vi "3-lorentzian-heat-response -- analytic derivatives -- grad and curvature -- V4.vi"(6 "parameters map  IN":map{T1, dbl}(c390), 7 "action":T2=enum."d-all", 10 "ω (rad/sec)":dbl=0.1 format="%#_10f") -> (0 "second derivatives map out":map{i32[], cdb}(c390), 1 "grad map  out":map{i32, cdb}(c390), 2 "ω out (rad/sec)":dbl=0.1 format="%#_10f", 3 "R(ω)":cdb=0.1+0.0i format="%#_10f")   [LabVIEW 2020]
uses:
  3-lorentzian-heat-response action.ctl
  3-lorentzian-parameters.ctl
panel:
  in  "κ0":dbl(slide)=6.091279771876994e-09 min=0.0 max=0.3 step=1e-12 scale=1e-10..1e-06 scale format="%#_3p"
  in  "ζ":dbl(slide)=0.016395386176563286 min=0.0 max=0.3 step=1e-06 scale=1e-05..1000.0 scale format="%#_3p"
  in  "τN":dbl(slide)=0.0007964886373917906 min=0.0 max=0.3 step=1e-06 scale=1e-06..10.0 scale format="%#_3p"
  in  "T1":dbl(slide)=0.017784241145719432 min=0.0 max=0.3 step=1e-06 scale=0.0001..10.0 scale format="%#_3p"
  in  "τC":dbl(slide)=0.0055481925503790405 min=0.0 max=0.3 step=1e-06 scale=0.0001..10.0 scale format="%#_3p"
  in  "τS":dbl(slide)=0.01833817297436167 min=0.0 max=0.3 step=1e-06 scale=0.0001..10.0 scale format="%#_3p"
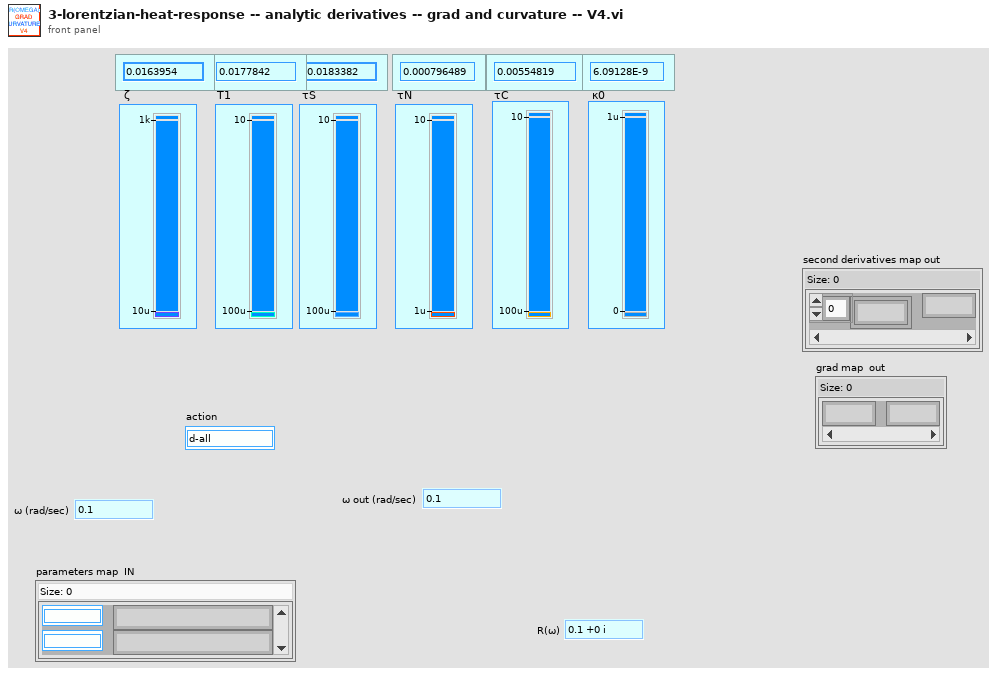
[diagram p1: front panel]
types:
  T1 = typedef "3-lorentzian-parameters.ctl" = enum16{"ζ", "τ1", "τS", "τN", "τC", "κ0", "m1", "m2", "m3", "T (K)", "B (T)", "θ (deg)", "side (S|R)", "set of (B|T)"}
  T2 = typedef "3-lorentzian-heat-response action.ctl" = enum16{"calc R", "create string", "calc m1m2m3", "dζ", "dT1", "dτS", "dτN", "dτC", "d-all", "dκ0", "T(K)", "m1", "m2", "m3", "parse string", "θ (deg)", "B (T)", "onlygrads", "newton", "create emty string"}
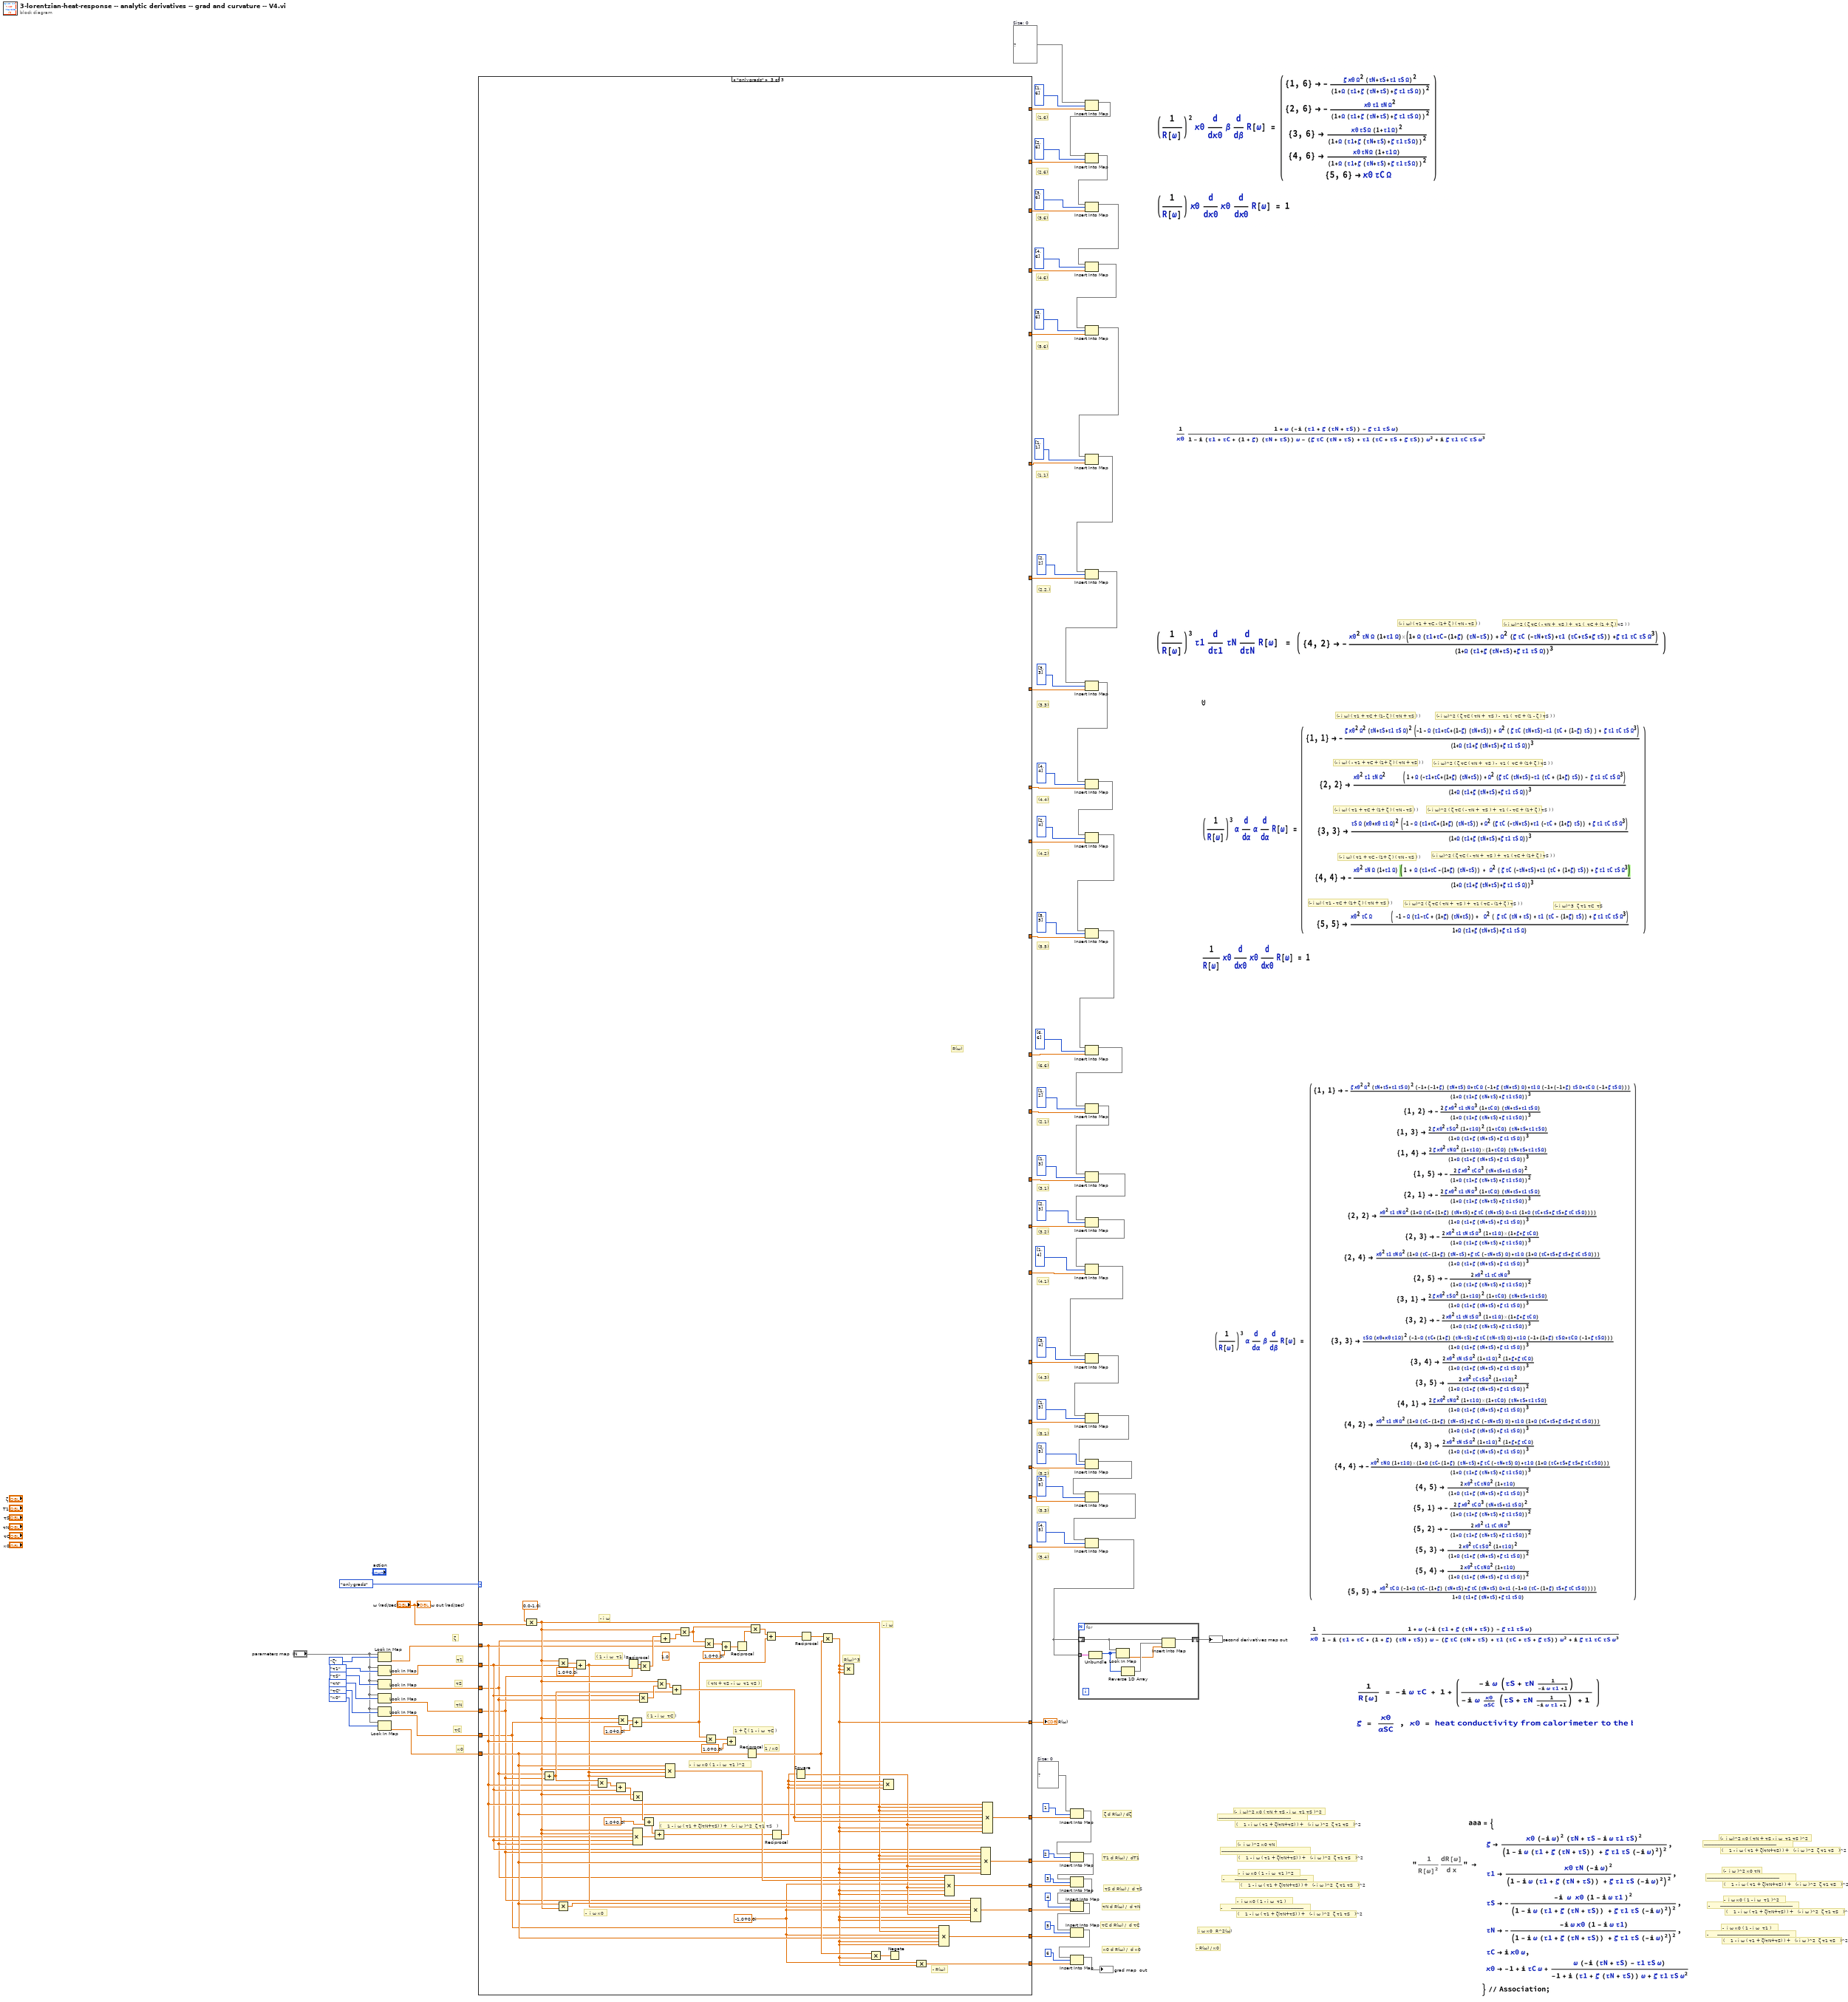
[diagram p0: block diagram]
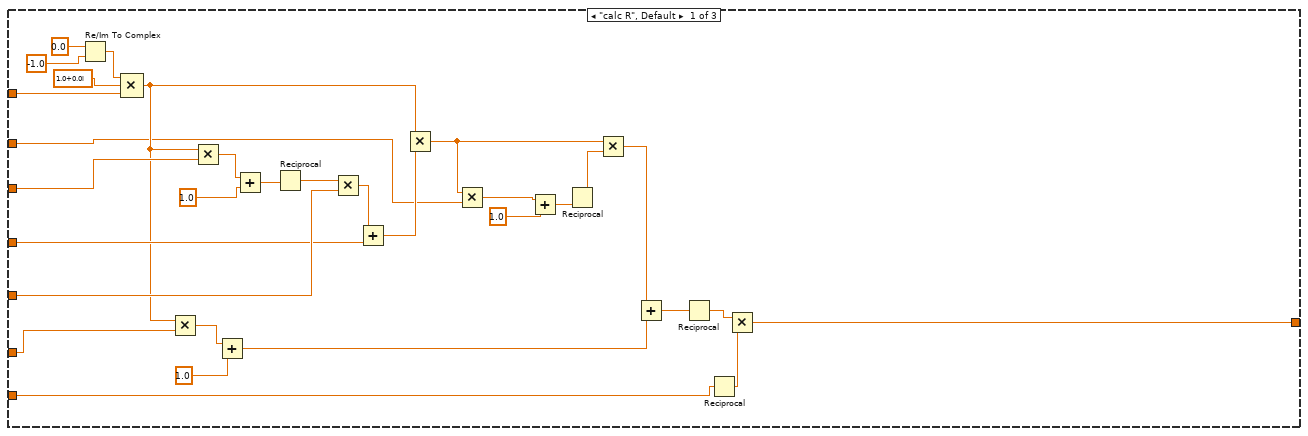
[diagram p2: hidden frame]
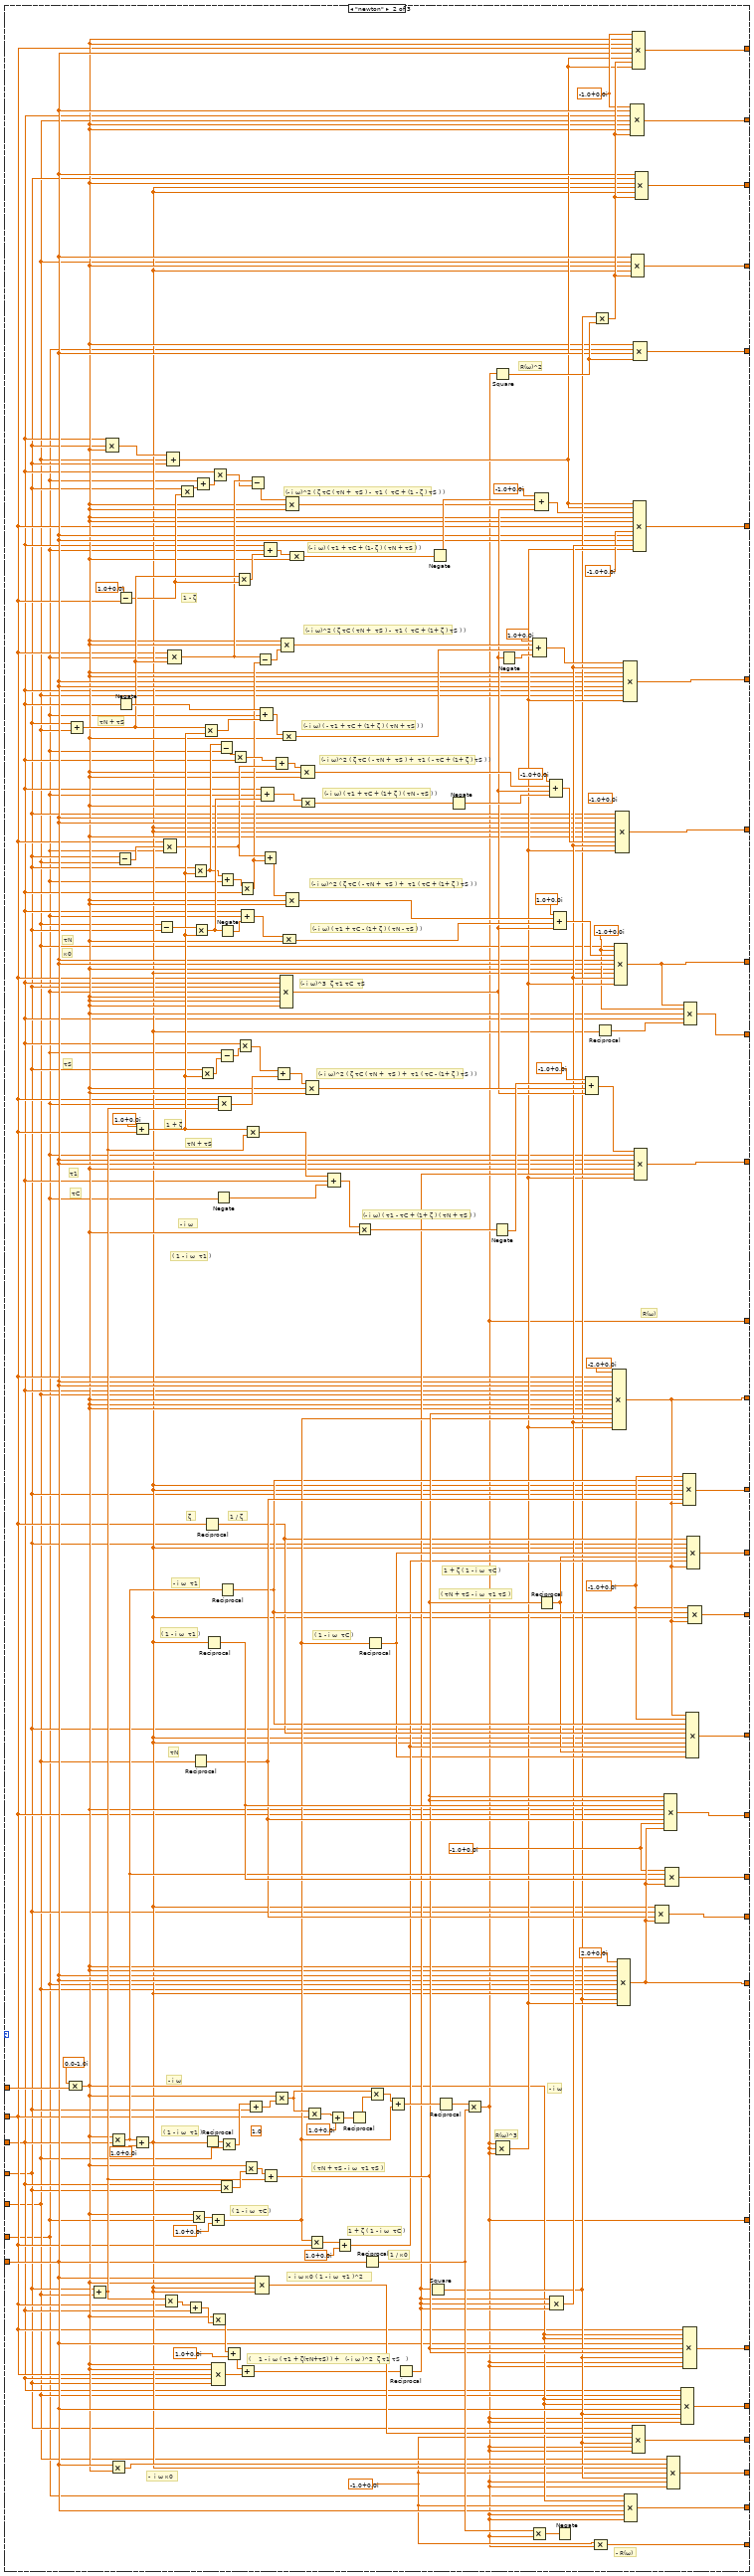
[diagram p3: hidden frame]
diagram:
  w27 = map{i32, cdb} {}  # Size: 0
  w85 = map{i32[], cdb} {}  # Size: 0
  # "κ0 d R(ω) /  d κ0"
  # "τC d R(ω) /  d τC"
  # "τN d R(ω) /  d τN"
  # "τS d R(ω) /  d τS"
  # "T1 d R(ω) /  dT1"
  # "ζ d R(ω) / dζ"
  # "(4,2)"
  # "(- i ω)^2 ( ζ τC ( - τN +  τS ) +  τ1 (  τC + (1 + ζ ) τS ) )"
  # "(- i ω) ( τ1 + τC - (1+ ζ ) ( τN - τS ) )"
  # "(1,6)"
  # "(2,6)"
  # "(3,6)"
  # "(4,6)"
  # "(5,6)"
  # "(1,1)"
  # "(- i ω)^2 ( ζ τC ( τN +  τS ) -  τ1 (  τC + (1 - ζ ) τS ) )"
  # "(- i ω) ( τ1 + τC + (1- ζ ) ( τN + τS ) )"
  # "(2,2,)"
  # "(- i ω)^2 ( ζ τC ( τN +  τS ) -  τ1 (  τC + (1+ ζ ) τS ) )"
  # "(- i ω) ( - τ1 + τC + (1+ ζ ) ( τN + τS ) )"
  # "(3,3)"
  # "(- i ω)^2 ( ζ τC ( - τN +  τS ) +  τ1 ( - τC + (1+ ζ ) τS ) )"
  # "(- i ω) ( τ1 + τC + (1+ ζ ) ( τN - τS ) )"
  # "(4,4)"
  # "(- i ω)^2 ( ζ τC ( - τN +  τS ) +  τ1 ( τC + (1+ ζ ) τS ) )"
  # "(- i ω) ( τ1 + τC - (1+ ζ ) ( τN - τS ) )"
  # "(- i ω)^3  ζ τ1 τC  τS"
  # "(- i ω) ( τ1 - τC + (1+ ζ ) ( τN + τS ) )"
  # "(- i ω)^2 ( ζ τC ( τN +  τS ) +  τ1 ( τC - (1+ ζ ) τS ) )"
  # "(5,5)"
  # "(6,6)"
  # "(4,3)"
  # "(4,1)"
  # "(3,2)"
  # "(3,1)"
  # "(2,1)"
  # "(5,1)"
  # "(5,2)"
  # "(5,3)"
  # "κ0"
  # "τC"
  # "τN"
  # "τS"
  # "τ1"
  # "ζ"
  # "(5,4)"
  # "-------------------------------------------------"
  # "(-  i ω)^2 κ0 ( τN + τS - i ω  τ1 τS )^2"
  # "(    1 - i ω ( τ1 + ζ(τN+τS) ) +   (- i ω )^2  ζ τ1 τS   )^2"
  # "-------------------------------------------------"
  # "(-  i ω )^2 κ0 τN"
  # "(    1 - i ω ( τ1 + ζ(τN+τS) ) +   (- i ω )^2  ζ τ1 τS   )^2"
  # "-      -------------------------------------------------"
  # "-  i ω κ0 ( 1 - i ω  τ1 )"
  # "(    1 - i ω ( τ1 + ζ(τN+τS) ) +   (- i ω )^2  ζ τ1 τS   )^2"
  # "-       -------------------------------------------------"
  # "-  i ω κ0 ( 1 - i ω  τ1 )^2"
  # "(    1 - i ω ( τ1 + ζ(τN+τS) ) +   (- i ω )^2  ζ τ1 τS   )^2"
  # "-------------------------------------------------"
  # "(-  i ω)^2 κ0 ( τN + τS - i ω  τ1 τS )^2"
  # "(    1 - i ω ( τ1 + ζ(τN+τS) ) +   (- i ω )^2  ζ τ1 τS   )^2"
  # "-------------------------------------------------"
  # "(-  i ω )^2 κ0 τN"
  # "(    1 - i ω ( τ1 + ζ(τN+τS) ) +   (- i ω )^2  ζ τ1 τS   )^2"
  # "-      -------------------------------------------------"
  # "-  i ω κ0 ( 1 - i ω  τ1 )"
  # "(    1 - i ω ( τ1 + ζ(τN+τS) ) +   (- i ω )^2  ζ τ1 τS   )^2"
  # "-       -------------------------------------------------"
  # "-  i ω κ0 ( 1 - i ω  τ1 )^2"
  # "(    1 - i ω ( τ1 + ζ(τN+τS) ) +   (- i ω )^2  ζ τ1 τS   )^2"
  # "i ω κ0  R^2(ω)"
  # "- R(ω) / κ0"
  n1 = Look In Map(map="parameters map  IN", key=3-lorentzian-parameters."ζ" ("Plost: sweep window")) -> (value=w91:dbl)  [unwired: 1 in, 1 out]
  n2 = Look In Map(map="parameters map  IN", key=3-lorentzian-parameters."τ1" ("Plost: sweep window")) -> (value=w90:dbl)  [unwired: 1 in, 1 out]
  n3 = Look In Map(map="parameters map  IN", key=3-lorentzian-parameters."τS" ("Plost: sweep window")) -> (value=w89:dbl)  [unwired: 1 in, 1 out]
  n4 = Look In Map(map="parameters map  IN", key=3-lorentzian-parameters."τN" ("Plost: sweep window")) -> (value=w88:dbl)  [unwired: 1 in, 1 out]
  n5 = Look In Map(map="parameters map  IN", key=3-lorentzian-parameters."τC" ("Plost: sweep window")) -> (value=w87:dbl)  [unwired: 1 in, 1 out]
  n6 = Look In Map(map="parameters map  IN", key=3-lorentzian-parameters."κ0" ("Plost: sweep window")) -> (value=w86:dbl)  [unwired: 1 in, 1 out]
  n7 = case shown="\"onlygrads\"" 3-lorentzian-heat-response_action."onlygrads" ("action") {
    tunnel: w87 -> [w117 w132 w289]
    tunnel: "ω (rad/sec)" -> [w120 w286 w339]
    tunnel: w90 -> [w119 w138 w295]
    tunnel: w88 -> [w125 w136 w293]
    tunnel: w89 -> [w123 w137 w294]
    tunnel: w91 -> [w113 w139 w296]
    tunnel: [w101 w134 w291] -> w100
    tunnel: w86 -> [w104 w148 w299]
    tunnel: [_ w133 w290] -> w10
    tunnel: [_ w274 w327] -> w14
    tunnel: [_ w263 w316] -> w20
    tunnel: [_ w261 w314] -> w16
    tunnel: [_ w260 w313] -> w23
    tunnel: [_ w257 w310] -> w25
    tunnel: [_ w251 _] -> w29
    tunnel: [_ w254 _] -> w31
    tunnel: [_ w253 _] -> w34
    tunnel: [_ w252 _] -> w37
    tunnel: [_ w237 _] -> w52
    tunnel: [_ w244 _] -> w49
    tunnel: [_ w239 _] -> w46
    tunnel: [_ w238 _] -> w43
    tunnel: [_ w236 _] -> w40
    tunnel: [_ w134 _] -> w56
    tunnel: [_ w214 _] -> w58
    tunnel: [_ w145 _] -> w60
    tunnel: [_ w194 _] -> w63
    tunnel: [_ w184 _] -> w66
    tunnel: [_ w160 _] -> w69
    tunnel: [_ w156 _] -> w71
    tunnel: [_ w153 _] -> w74
    tunnel: [_ w152 _] -> w78
    tunnel: [_ w151 _] -> w80
    tunnel: [_ w147 _] -> w83
    tunnel: [_ w140 _] -> w3
    frame "calc R", Default {
      n8 = Re/Im To Complex(1:-1.0 ("y"), 2:0.0 ("x")) -> (0:w121:cdb)
      n9 = Compound Arithmetic op=MULTIPLY(w121, cdb 1.0+0.0i ("value"), w120) -> (w115:cdb)
      n10 = Multiply(x=w115, y=w117) -> (x*y=w116:cdb)
      n11 = Multiply(x=w115, y=w119) -> (x*y=w118:cdb)
      n12 = Add(x=w116, y=1.0) -> (x+y=w107:cdb)
      n13 = Add(x=w118, y=1.0) -> (x+y=w127:cdb)
      n14 = Reciprocal(x=w127) -> (1/x=w126:cdb)
      n15 = Multiply(x=w126, y=w125) -> (x*y=w124:cdb)
      n16 = Add(x=w124, y=w123) -> (x+y=w114:cdb)
      n17 = Multiply(x=w115, y=w114) -> (x*y=w109:cdb)
      n18 = Multiply(x=w109, y=w113) -> (x*y=w111:cdb)
      n19 = Add(x=w111, y=1.0) -> (x+y=w110:cdb)
      n20 = Reciprocal(x=w110) -> (1/x=w108:cdb)
      n21 = Multiply(x=w109, y=w108) -> (x*y=w106:cdb)
      n22 = Add(x=w106, y=w107) -> (x+y=w105:cdb)
      n23 = Reciprocal(x=w105) -> (1/x=w103:cdb)
      n24 = Reciprocal(x=w104) -> (1/x=w102:dbl)
      n25 = Multiply(x=w103, y=w102) -> (x*y=w101:cdb)
    }
    frame "newton" {
      w149 = cdb -1.0+0.0i ("value")
      (unwired) cdb -1.0+0.0i ("value")
      w144 = cdb -1.0+0.0i ("value")
      w235 = cdb -1.0+0.0i ("value")
      w250 = cdb -1.0+0.0i ("value")
      w135 = cdb -1.0+0.0i ("value")
      (unwired) 1.0
      # "(- i ω)^2 ( ζ τC ( τN +  τS ) -  τ1 (  τC + (1 - ζ ) τS ) )"
      # "(- i ω) ( τ1 + τC + (1- ζ ) ( τN + τS ) )"
      # "τN + τS"
      # "(- i ω)^2 ( ζ τC ( τN +  τS ) -  τ1 (  τC + (1+ ζ ) τS ) )"
      # "(- i ω) ( - τ1 + τC + (1+ ζ ) ( τN + τS ) )"
      # "(- i ω)^2 ( ζ τC ( - τN +  τS ) +  τ1 ( - τC + (1+ ζ ) τS ) )"
      # "(- i ω) ( τ1 + τC + (1+ ζ ) ( τN - τS ) )"
      # "κ0"
      # "τN"
      # "( 1 - i ω  τ1 )"
      # "(- i ω)^2 ( ζ τC ( - τN +  τS ) +  τ1 ( τC + (1+ ζ ) τS ) )"
      # "(- i ω) ( τ1 + τC - (1+ ζ ) ( τN - τS ) )"
      # "τS"
      # "τ1"
      # "(- i ω)^3  ζ τ1 τC  τS"
      # "(- i ω)^2 ( ζ τC ( τN +  τS ) +  τ1 ( τC - (1+ ζ ) τS ) )"
      # "1 - ζ"
      # "(- i ω) ( τ1 - τC + (1+ ζ ) ( τN + τS ) )"
      # "- i ω"
      # "τC"
      # "τN + τS"
      # "1 + ζ"
      # "R(ω)"
      # "τN"
      # "1 / ζ"
      # "ζ"
      # "- i ω  τ1"
      # "( 1 - i ω  τ1 )"
      # "( τN + τS - i ω  τ1 τS )"
      # "1 + ζ ( 1 - i ω  τC )"
      # "( 1 - i ω  τC )"
      # "1 + ζ ( 1 - i ω  τC )"
      # "( 1 - i ω  τC )"
      # "R(ω)^3"
      # "( τN + τS - i ω  τ1 τS )"
      # "-  i ω κ0"
      # "( 1 - i ω  τ1 )"
      # "(    1 - i ω ( τ1 + ζ(τN+τS) ) +   (- i ω )^2  ζ τ1 τS   )"
      # "-  i ω κ0 ( 1 - i ω  τ1 )^2"
      # "- i ω"
      # "1 / κ0"
      # "- R(ω)"
      # "- i ω"
      # "R(ω)^2"
      n26 = Add(x=w137, y=w136) -> (x+y=w182:dbl)
      n27 = Compound Arithmetic op=MULTIPLY(cdb 0.0-1.0i ("value"), w286) -> (w143:cdb)
      n28 = Add(x=w137, y=w136) -> (x+y=w225:dbl)
      n29 = Compound Arithmetic op=MULTIPLY(w138, w137, w143) -> (w159:cdb)
      n30 = Multiply(x=w143, y=w138) -> (x*y=w246:cdb)
      n31 = Multiply(x=w148, y=w143) -> (x*y=w262:cdb)
      n32 = Subtract(x=w137, y=w136) -> (x-y=w209:dbl)
      n33 = Subtract(x=cdb 1.0+0.0i ("value"), y=w139) -> (x-y=w173:cdb)
      n34 = Negate(x=w138) -> (-x=w192:dbl)
      n35 = Add(x=cdb 1.0+0.0i ("value"), y=w139) -> (x+y=w193:cdb)
      n36 = Add(x=w246, y=cdb 1.0+0.0i ("value")) -> (x+y=w142:cdb)
      n37 = Subtract(x=w136, y=w137) -> (x-y=w212:dbl)
      n38 = Multiply(x=w225, y=w139) -> (x*y=w270:dbl)
      n39 = Compound Arithmetic op=MULTIPLY(w139, w209, w132) -> (w200:dbl)
      n40 = Compound Arithmetic op=ADD(w159, w136, w137) -> (w146:cdb)
      n41 = Compound Arithmetic op=MULTIPLY(w139, w132, w182) -> (w170:dbl)
      n42 = Multiply(x=w137, y=w173) -> (x*y=w172:cdb)
      n43 = Add(x=w270, y=w138) -> (x+y=w269:dbl)
      n44 = Multiply(x=w143, y=w132) -> (x*y=w285:cdb)
      n45 = Multiply(x=w137, y=w193) -> (x*y=w203:cdb)
      n46 = Reciprocal(x=w136) -> (1/x=w245:dbl)
      n47 = Multiply(x=w212, y=w193) -> (x*y=w204:cdb)
      n48 = Add(x=w132, y=w172) -> (x+y=w171:cdb)
      n49 = Multiply(x=w137, y=w193) -> (x*y=w224:cdb)
      n50 = Multiply(x=w182, y=w193) -> (x*y=w191:cdb)
      n51 = Reciprocal(x=w139) -> (1/x=w233:dbl)
      n52 = Reciprocal(x=w142) -> (1/x=w288:cdb)
      n53 = Reciprocal(x=w142) -> (1/x=w247:cdb)
      n54 = Add(x=w285, y=cdb 1.0+0.0i ("value")) -> (x+y=w242:cdb)
      n55 = Multiply(x=w143, y=w269) -> (x*y=w268:cdb)
      n56 = Multiply(x=w138, y=w171) -> (x*y=w169:cdb)
      n57 = Compound Arithmetic op=MULTIPLY(w143, w143, w139, w138, w137) -> (w265:cdb)
      n58 = Negate(x=w132) -> (-x=w228:dbl)
      n59 = Subtract(x=w203, y=w132) -> (x-y=w202:cdb)
      n60 = Multiply(x=w138, y=w137) -> (x*y=w259:dbl)
      n61 = Subtract(x=w132, y=w224) -> (x-y=w223:cdb)
      n62 = Compound Arithmetic op=MULTIPLY(w139, w132, w225) -> (w221:dbl)
      n63 = Add(x=w203, y=w132) -> (x+y=w210:cdb)
      n64 = Negate(x=w204) -> (-x=w211:cdb)
      n65 = Reciprocal(x=w246) -> (1/x=w234:cdb)
      n66 = Multiply(x=w288, y=w136) -> (x*y=w287:cdb)
      n67 = Add(x=w268, y=cdb 1.0+0.0i ("value")) -> (x+y=w266:cdb)
      n68 = Multiply(x=w202, y=w138) -> (x*y=w201:cdb)
      n69 = Multiply(x=w182, y=w173) -> (x*y=w181:cdb)
      n70 = Multiply(x=w138, y=w223) -> (x*y=w222:cdb)
      n71 = Multiply(x=w210, y=w138) -> (x*y=w189:cdb)
      n72 = Add(x=w266, y=w265) -> (x+y=w248:cdb)
      n73 = Compound Arithmetic op=ADD(w138, w132, w211) -> (w175:cdb)
      n74 = Multiply(x=w143, y=w259) -> (x*y=w258:cdb)
      n75 = Multiply(x=w193, y=w225) -> (x*y=w229:cdb)
      n76 = Add(x=w287, y=w137) -> (x+y=w284:cdb)
      n77 = Subtract(x=w170, y=w169) -> (x-y=w168:cdb)
      n78 = Compound Arithmetic op=MULTIPLY(w148, w143, w142, w142) -> (w264:cdb)
      n79 = Subtract(x=w170, y=w189) -> (x-y=w179:cdb)
      n80 = Compound Arithmetic op=ADD(w192, w132, w191) -> (w190:cdb)
      n81 = Compound Arithmetic op=ADD(w138, w132, w204) -> (w177:cdb)
      n82 = Add(x=w200, y=w189) -> (x+y=w208:cdb)
      n83 = Add(x=w258, y=w225) -> (x+y=w243:cdb)
      n84 = Compound Arithmetic op=ADD(w138, w132, w181) -> (w180:cdb)
      n85 = Add(x=w201, y=w200) -> (x+y=w199:cdb)
      n86 = Multiply(x=w143, y=w284) -> (x*y=w281:cdb)
      n87 = Add(x=w222, y=w221) -> (x+y=w220:cdb)
      n88 = Compound Arithmetic op=MULTIPLY(w139, w138, w137, w132, w143, w143, w143) -> (w163:cdb)
      n89 = Compound Arithmetic op=MULTIPLY(w143, w143, w179) -> (w178:cdb)
      n90 = Compound Arithmetic op=MULTIPLY(w190, w143) -> (w187:cdb)
      n91 = Compound Arithmetic op=MULTIPLY(w175, w143) -> (w174:cdb)
      n92 = Compound Arithmetic op=MULTIPLY(w168, w143, w143) -> (w164:cdb)
      n93 = Compound Arithmetic op=MULTIPLY(w208, w143, w143) -> (w206:cdb)
      n94 = Compound Arithmetic op=MULTIPLY(w180, w143) -> (w166:cdb)
      n95 = Compound Arithmetic op=MULTIPLY(w199, w143, w143) -> (w197:cdb)
      n96 = Compound Arithmetic op=MULTIPLY(w177, w143) -> (w176:cdb)
      n97 = Compound Arithmetic op=MULTIPLY(w220, w143, w143) -> (w216:cdb)
      n98 = Multiply(x=w281, y=w139) -> (x*y=w283:cdb)
      n99 = Multiply(x=w242, y=w139) -> (x*y=w241:cdb)
      n100 = Compound Arithmetic op=ADD(w229, w138, w228) -> (w227:cdb)
      n101 = Add(x=w283, y=cdb 1.0+0.0i ("value")) -> (x+y=w282:cdb)
      n102 = Add(x=w241, y=cdb 1.0+0.0i ("value")) -> (x+y=w232:cdb)
      n103 = Reciprocal(x=w282) -> (1/x=w280:cdb)
      n104 = Multiply(x=w227, y=w143) -> (x*y=w219:cdb)
      n105 = Reciprocal(x=w148) -> (1/x=w276:dbl)
      n106 = Reciprocal(x=w242) -> (1/x=w230:cdb)
      n107 = Multiply(x=w281, y=w280) -> (x*y=w279:cdb)
      n108 = Add(x=w279, y=w242) -> (x+y=w278:cdb)
      n109 = Reciprocal(x=w248) -> (1/x=w213:cdb)
      n110 = Square(x=w213) -> (x^2=w154:cdb)
      n111 = Negate(x=w166) -> (-x=w165:cdb)
      n112 = Reciprocal(x=w278) -> (1/x=w277:cdb)
      n113 = Negate(x=w176) -> (-x=w196:cdb)
      n114 = Multiply(x=w277, y=w276) -> (x*y=w134:cdb)
      n115 = Negate(x=w219) -> (-x=w217:cdb)
      n116 = Square(x=w134) -> (x^2=w155:cdb)
      n117 = Compound Arithmetic op=MULTIPLY(w134, w134, w134) -> (w157:cdb)
      n118 = Negate(x=w163) -> (-x=w186:cdb)
      n119 = Multiply(x=w276, y=w134) -> (x*y=w275:cdb)
      n120 = Compound Arithmetic op=ADD(cdb 1.0+0.0i ("value"), w178, w187, w186) -> (w185:cdb)
      n121 = Compound Arithmetic op=ADD(cdb -1.0+0.0i ("value"), w165, w164, w163) -> (w162:cdb)
      n122 = Reciprocal(x=w243) -> (1/x=w231:cdb)
      n123 = Compound Arithmetic op=ADD(cdb -1.0+0.0i ("value"), w197, w163, w196) -> (w195:cdb)
      n124 = Compound Arithmetic op=MULTIPLY(w213, w213, w213) -> (w161:cdb)
      n125 = Compound Arithmetic op=ADD(cdb 1.0+0.0i ("value"), w206, w174, w163) -> (w205:cdb)
      n126 = Negate(x=w275) -> ()  [unwired: 1 out]
      n127 = Compound Arithmetic op=ADD(cdb -1.0+0.0i ("value"), w217, w216, w163) -> (w215:cdb)
      n128 = Multiply(x=w154, y=w155) -> (x*y=w150:cdb)
      n129 = Compound Arithmetic op=MULTIPLY(w135, w134) -> (w133:cdb)
      n130 = Reciprocal(x=w142) -> (1/x=w141:cdb)
      n131 = Compound Arithmetic op=MULTIPLY(cdb -2.0+0.0i ("value"), w139, w148, w148, w138, w136, w143, w143, w143, w243, w242, w161, w157) -> (w237:cdb)
      n132 = Compound Arithmetic op=MULTIPLY(w136, w144, w205, w148, w148, w143, w142, w161, w157) -> (w145:cdb)
      n133 = Compound Arithmetic op=MULTIPLY(w137, w148, w148, w142, w142, w143, w195, w161, w157) -> (w194:cdb)
      n134 = Compound Arithmetic op=MULTIPLY(cdb 2.0+0.0i ("value"), w143, w143, w148, w148, w132, w136, w142, w154, w157) -> (w251:cdb)
      n135 = Compound Arithmetic op=MULTIPLY(w185, w161, w143, w143, w148, w148, w138, w136, w157) -> (w184:cdb)
      n136 = Compound Arithmetic op=MULTIPLY(w132, w143, w135, w148, w134, w134) -> (w274:cdb)
      n137 = Compound Arithmetic op=MULTIPLY(w149, w148, w138, w136, w143, w143, w150) -> (w151:cdb)
      n138 = Compound Arithmetic op=MULTIPLY(w148, w136, w143, w142, w150) -> (w153:cdb)
      n139 = Compound Arithmetic op=MULTIPLY(w149, w143, w143, w139, w148, w146, w150, w146) -> (w147:cdb)
      n140 = Compound Arithmetic op=MULTIPLY(w137, w264, w135, w154, w134, w134) -> (w263:cdb)
      n141 = Compound Arithmetic op=MULTIPLY(w146, w146, w162, w143, w143, w139, cdb -1.0+0.0i ("value"), w148, w148, w161, w157) -> (w160:cdb)
      n142 = Compound Arithmetic op=MULTIPLY(w143, w132, w148, w155) -> (w156:cdb)
      n143 = Compound Arithmetic op=MULTIPLY(w215, w132, w148, w148, w143, w213, w157) -> (w214:cdb)
      n144 = Compound Arithmetic op=MULTIPLY(w148, w137, w143, w142, w142, w150) -> (w152:cdb)
      n145 = Compound Arithmetic op=MULTIPLY(w142, w137, w245, w251) -> (w254:cdb)
      n146 = Compound Arithmetic op=MULTIPLY(w243, w243, w247, w143, w139, w245, w250, w251) -> (w252:cdb)
      n147 = Compound Arithmetic op=MULTIPLY(w250, w246, w247, w251) -> (w253:cdb)
      n148 = Compound Arithmetic op=MULTIPLY(w136, w262, w142, w135, w154, w134, w134) -> (w261:cdb)
      n149 = Compound Arithmetic op=MULTIPLY(w138, w136, w143, w143, w148, w154, w134, w134) -> (w260:cdb)
      n150 = Compound Arithmetic op=MULTIPLY(w235, w234, w142, w142, w137, w245, w237) -> (w244:cdb)
      n151 = Compound Arithmetic op=MULTIPLY(w139, w143, w143, w148, w243, w243, w154, w134, w134) -> (w257:cdb)
      n152 = Compound Arithmetic op=MULTIPLY(w145, w144, w143, w138, w141) -> (w140:cdb)
      n153 = Compound Arithmetic op=MULTIPLY(w237, w235, w234, w137, w233, w142, w142, w232, w231, w230) -> (w236:cdb)
      n154 = Compound Arithmetic op=MULTIPLY(w233, w137, w142, w230, w231, w232, w237) -> (w239:cdb)
      n155 = Compound Arithmetic op=MULTIPLY(w235, w234, w142, w237) -> (w238:cdb)
    }
    frame "onlygrads" {
      w292 = cdb -1.0+0.0i ("value")
      (unwired) 1.0
      # "R(ω)"
      # "1 + ζ ( 1 - i ω  τC )"
      # "( 1 - i ω  τC )"
      # "R(ω)^3"
      # "( τN + τS - i ω  τ1 τS )"
      # "-  i ω κ0"
      # "( 1 - i ω  τ1 )"
      # "(    1 - i ω ( τ1 + ζ(τN+τS) ) +   (- i ω )^2  ζ τ1 τS   )"
      # "-  i ω κ0 ( 1 - i ω  τ1 )^2"
      # "- i ω"
      # "1 / κ0"
      # "- R(ω)"
      # "- i ω"
      n156 = Compound Arithmetic op=MULTIPLY(cdb 0.0-1.0i ("value"), w339) -> (w298:cdb)
      n157 = Add(x=w294, y=w293) -> (x+y=w302:dbl)
      n158 = Multiply(x=w298, y=w295) -> (x*y=w307:cdb)
      n159 = Multiply(x=w299, y=w298) -> (x*y=w315:cdb)
      n160 = Add(x=w307, y=cdb 1.0+0.0i ("value")) -> (x+y=w297:cdb)
      n161 = Multiply(x=w302, y=w296) -> (x*y=w323:dbl)
      n162 = Add(x=w323, y=w295) -> (x+y=w322:dbl)
      n163 = Multiply(x=w298, y=w289) -> (x*y=w338:cdb)
      n164 = Reciprocal(x=w297) -> (1/x=w341:cdb)
      n165 = Add(x=w338, y=cdb 1.0+0.0i ("value")) -> (x+y=w305:cdb)
      n166 = Multiply(x=w298, y=w322) -> (x*y=w321:cdb)
      n167 = Compound Arithmetic op=MULTIPLY(w298, w298, w296, w295, w294) -> (w318:cdb)
      n168 = Multiply(x=w295, y=w294) -> (x*y=w312:dbl)
      n169 = Multiply(x=w341, y=w293) -> (x*y=w340:cdb)
      n170 = Add(x=w321, y=cdb 1.0+0.0i ("value")) -> (x+y=w319:cdb)
      n171 = Add(x=w319, y=w318) -> (x+y=w308:cdb)
      n172 = Multiply(x=w298, y=w312) -> (x*y=w311:cdb)
      n173 = Add(x=w340, y=w294) -> (x+y=w337:cdb)
      n174 = Compound Arithmetic op=MULTIPLY(w299, w298, w297, w297) -> (w317:cdb)
      n175 = Add(x=w311, y=w302) -> (x+y=w306:cdb)
      n176 = Multiply(x=w298, y=w337) -> (x*y=w334:cdb)
      n177 = Multiply(x=w334, y=w296) -> (x*y=w336:cdb)
      n178 = Multiply(x=w305, y=w296) -> (x*y=w304:cdb)
      n179 = Add(x=w336, y=cdb 1.0+0.0i ("value")) -> (x+y=w335:cdb)
      n180 = Add(x=w304, y=cdb 1.0+0.0i ("value")) -> ()  [unwired: 1 out]
      n181 = Reciprocal(x=w335) -> (1/x=w333:cdb)
      n182 = Reciprocal(x=w299) -> (1/x=w329:dbl)
      n183 = Multiply(x=w334, y=w333) -> (x*y=w332:cdb)
      n184 = Add(x=w332, y=w305) -> (x+y=w331:cdb)
      n185 = Reciprocal(x=w308) -> (1/x=w301:cdb)
      n186 = Square(x=w301) -> (x^2=w300:cdb)
      n187 = Reciprocal(x=w331) -> (1/x=w330:cdb)
      n188 = Multiply(x=w330, y=w329) -> (x*y=w291:cdb)
      n189 = Compound Arithmetic op=MULTIPLY(w291, w291, w291) -> ()  [unwired: 1 out]
      n190 = Multiply(x=w329, y=w291) -> (x*y=w328:cdb)
      n191 = Compound Arithmetic op=MULTIPLY(w301, w301, w301) -> ()  [unwired: 1 out]
      n192 = Negate(x=w328) -> ()  [unwired: 1 out]
      n193 = Compound Arithmetic op=MULTIPLY(w292, w291) -> (w290:cdb)
      n194 = Compound Arithmetic op=MULTIPLY(w289, w298, w292, w299, w291, w291) -> (w327:cdb)
      n195 = Compound Arithmetic op=MULTIPLY(w294, w317, w292, w300, w291, w291) -> (w316:cdb)
      n196 = Compound Arithmetic op=MULTIPLY(w293, w315, w297, w292, w300, w291, w291) -> (w314:cdb)
      n197 = Compound Arithmetic op=MULTIPLY(w295, w293, w298, w298, w299, w300, w291, w291) -> (w313:cdb)
      n198 = Compound Arithmetic op=MULTIPLY(w296, w298, w298, w299, w306, w306, w300, w291, w291) -> (w310:cdb)
    }
  }
  "R(ω)" <- w100
  n199 = Insert Into Map(map in=w27, key=1, value=w25) -> (map out=w24:map{i32, cdb})  [unwired: 2 out]
  n200 = Insert Into Map(map in=w24, key=2, value=w23) -> (map out=w21:map{i32, cdb})  [unwired: 2 out]
  n201 = Insert Into Map(map in=w21, key=3, value=w20) -> (map out=w18:map{i32, cdb})  [unwired: 2 out]
  n202 = Insert Into Map(map in=w18, key=4, value=w16) -> (map out=w15:map{i32, cdb})  [unwired: 2 out]
  n203 = Insert Into Map(map in=w15, key=5, value=w14) -> (map out=w12:map{i32, cdb})  [unwired: 2 out]
  n204 = Insert Into Map(map in=w12, key=6, value=w10) -> (map out=→"grad map  out":map{i32, cdb})  [unwired: 2 out]
  n205 = Insert Into Map(map in=w85, key=i32[] [1, 6], value=w83) -> (map out=w82:map{i32[], cdb})  [unwired: 2 out]
  n206 = Insert Into Map(map in=w82, key=i32[] [2, 6], value=w80) -> (map out=w79:map{i32[], cdb})  [unwired: 2 out]
  n207 = Insert Into Map(map in=w79, key=i32[] [3, 6], value=w78) -> (map out=w75:map{i32[], cdb})  [unwired: 2 out]
  n208 = Insert Into Map(map in=w75, key=i32[] [4, 6], value=w74) -> (map out=w72:map{i32[], cdb})  [unwired: 2 out]
  n209 = Insert Into Map(map in=w72, key=i32[] [5, 6], value=w71) -> (map out=w70:map{i32[], cdb})  [unwired: 2 out]
  n210 = Insert Into Map(map in=w70, key=i32[] [1, 1], value=w69) -> (map out=w67:map{i32[], cdb})  [unwired: 2 out]
  n211 = Insert Into Map(map in=w67, key=i32[] [2, 2], value=w66) -> (map out=w64:map{i32[], cdb})  [unwired: 2 out]
  n212 = Insert Into Map(map in=w64, key=i32[] [3, 3], value=w63) -> (map out=w61:map{i32[], cdb})  [unwired: 2 out]
  n213 = Insert Into Map(map in=w61, key=i32[] [4, 4], value=w60) -> (map out=w5:map{i32[], cdb})  [unwired: 2 out]
  n214 = Insert Into Map(map in=w5, key=i32[] [2, 4], value=w3) -> (map out=w4:map{i32[], cdb})  [unwired: 2 out]
  n215 = Insert Into Map(map in=w4, key=i32[] [5, 5], value=w58) -> (map out=w55:map{i32[], cdb})  [unwired: 2 out]
  n216 = Insert Into Map(map in=w55, key=i32[] [6, 6], value=w56) -> (map out=w53:map{i32[], cdb})  [unwired: 2 out]
  n217 = Insert Into Map(map in=w53, key=i32[] [1, 2], value=w52) -> (map out=w50:map{i32[], cdb})  [unwired: 2 out]
  n218 = Insert Into Map(map in=w50, key=i32[] [1, 3], value=w49) -> (map out=w47:map{i32[], cdb})  [unwired: 2 out]
  n219 = Insert Into Map(map in=w47, key=i32[] [2, 3], value=w46) -> (map out=w44:map{i32[], cdb})  [unwired: 2 out]
  n220 = Insert Into Map(map in=w44, key=i32[] [1, 4], value=w43) -> (map out=w41:map{i32[], cdb})  [unwired: 2 out]
  n221 = Insert Into Map(map in=w41, key=i32[] [3, 4], value=w40) -> (map out=w38:map{i32[], cdb})  [unwired: 2 out]
  n222 = Insert Into Map(map in=w38, key=i32[] [1, 5], value=w37) -> (map out=w35:map{i32[], cdb})  [unwired: 2 out]
  n223 = Insert Into Map(map in=w35, key=i32[] [2, 5], value=w34) -> (map out=w32:map{i32[], cdb})  [unwired: 2 out]
  n224 = Insert Into Map(map in=w32, key=i32[] [3, 5], value=w31) -> (map out=w28:map{i32[], cdb})  [unwired: 2 out]
  n225 = Insert Into Map(map in=w28, key=i32[] [4, 5], value=w29) -> (map out=w8:map{i32[], cdb})  [unwired: 2 out]
  n226 = for {
    tunnel: w8 -> [w347] mode=indexing
    shift-right: [w345] -> w7
    shift-left: w8 -> [w346]
    n227 = Unbundle(w347) -> (w344:i32[])  [unwired: 1 out]
    n228 = Look In Map(map=w346, key=w344) -> (value=w342:cdb)  [unwired: 1 in, 1 out]
    n229 = Reverse 1D Array(array=w344) -> (reversed array=w343:i32[])
    n230 = Insert Into Map(map in=w346, key=w343, value=w342) -> (map out=w345:map{i32[], cdb})  [unwired: 2 out]
  }
  "second derivatives map out" <- w7
  "ω out (rad/sec)" <- "ω (rad/sec)"
